vi "Read BallonTipText.vi"(8 "error in (no error)":errorcluster, 11 "BalloonTip in":refnum<class "BalloonTip.lvclass">) -> (0 "error out":errorcluster, 2 "BallonTipText":string, 3 "BalloonTip out":refnum<class "BalloonTip.lvclass">)   [LabVIEW 2016, in "BalloonTip.lvclass"]
uses:
  BalloonTip.lvclass
  BalloonTip.lvclass/BalloonTip.ctl
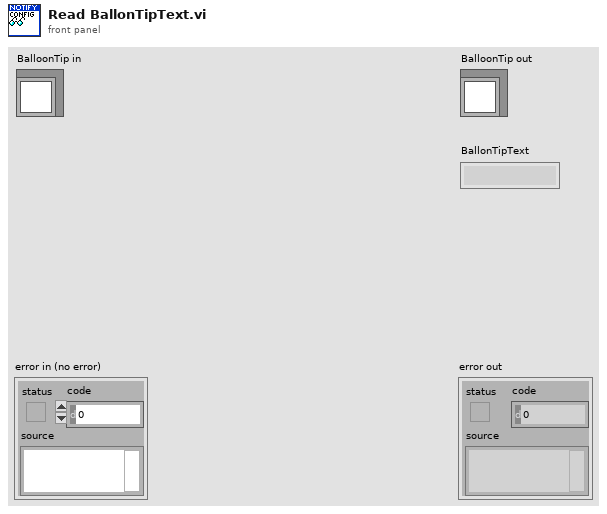
[diagram p1: front panel]
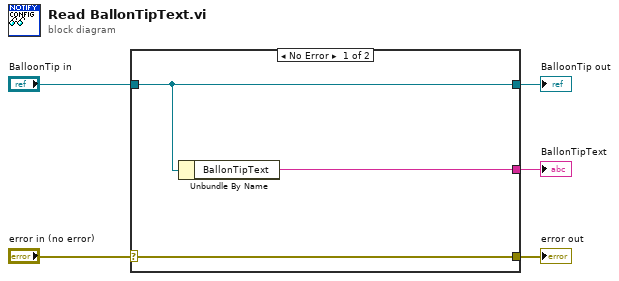
[diagram p0: block diagram]
diagram:
  n1 = case shown="No Error" "error in (no error)" {
    selector: "error in (no error)" -> [w8 w9]
    tunnel: [w8 w9] -> w4
    tunnel: [w7 w10] -> w2
    tunnel: "BalloonTip in" -> [w7 w10]
    tunnel: [w6 _] -> w1
    frame No Error {
      n2 = Unbundle By Name(w7) -> ("BallonTipText"=w6:string)
    }
    frame Error {
    }
  }
  "error out" <- w4
  "BalloonTip out" <- w2
  "BallonTipText" <- w1
